vi "Get Children.vi"(8 "error in (no error)":errorcluster, 10 "All Data":refnum<class "Data Item.lvclass">[](array[class]), 11 "Element in":refnum<class "Element.lvclass">) -> (0 "error out":errorcluster, 1 "Children Indices":i32[](array[numeric]), 2 "Children":refnum<class "Data Item.lvclass">[](array[class]), 3 "Element out":refnum<class "Element.lvclass">)   [LabVIEW 2026, in "VILab.lvlib" / "Element.lvclass"]
uses:
  Element.lvclass
  Data Item/Data Item.lvclass
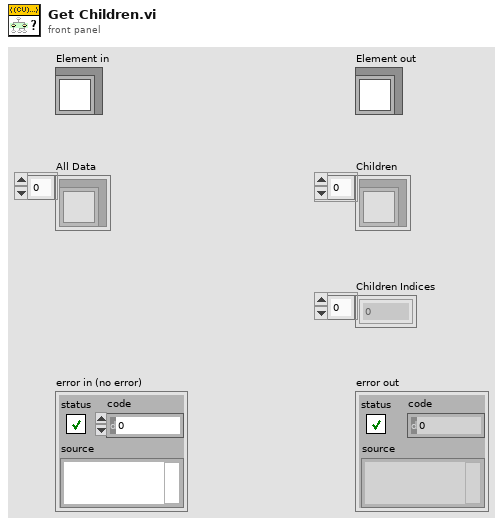
[diagram p1: front panel]
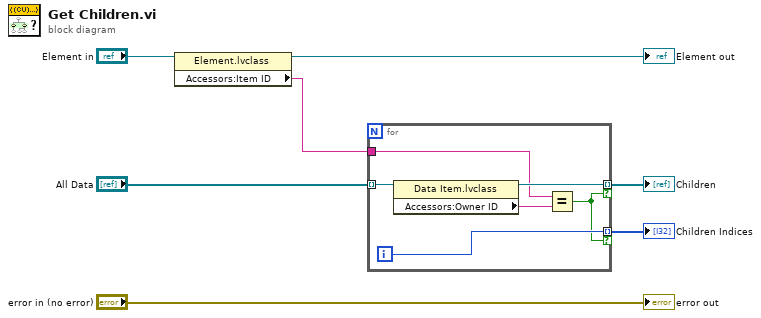
[diagram p0: block diagram]
diagram:
  n1 = property class="Element.lvclass"(reference="Element in") -> (reference out=→"Element out":refnum<class "Element.lvclass">, "Accessors:Item ID"=w4:string)  [unwired: 1 in, 1 out]
  n2 = for {
    tunnel: "All Data" -> [w13] mode=indexing
    tunnel: w4 -> [w10]
    tunnel: [w12] -> w3 mode=indexing if=w8
    tunnel: [w9] -> w1 mode=indexing if=w8
    i -> [w9]
    n3 = property class="Data Item.lvclass"(reference=w13) -> (reference out=w12:refnum<class "Data Item.lvclass">, "Accessors:Owner ID"=w11:string)  [unwired: 1 in, 1 out]
    n4 = Equal?(x=w10, y=w11) -> (x = y?=w8:bool)
  }
  "Children" <- w3
  "Children Indices" <- w1
  "error out" <- "error in (no error)"
